vi "Setup Log.vi"(0 "reference in":refnum<class "Result Logger.lvclass">, 4 "Logger Save Folder Path":path, 5 "error in (no error)":errorcluster, 7 "File Column Headers":string[](array[string])) -> (14 "reference out":refnum<class "Result Logger.lvclass">, 19 "error out":errorcluster)   [LabVIEW 2017, in "Result Logger.lvclass"]
uses:
  Result Logger.lvclass
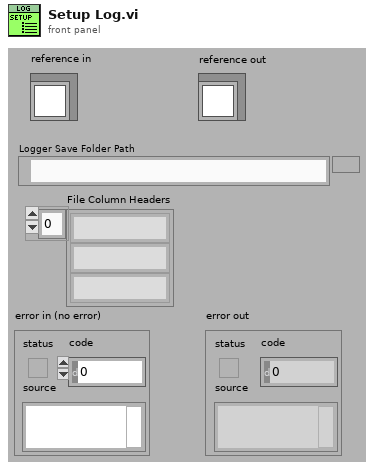
[diagram p1: front panel]
types:
  T1 = enum16{"open", "replace", "create", "open or create", "replace or create", "replace or create with confirmation"}
  T2 = typedef "Result Logger.lvclass/ObjectAttributes.ctl" = cluster{"Logger File Path":path, "Logger File Stream":refnum<file>, "Log Messages":T3[]}
  T3 = typedef "Result Logger.lvclass/Message.ctl" = cluster{"UUT Info":cluster{"Part Number":string, "Lower Push Limit (lb)":dbl, "Upper Push Limit (lb)":dbl, "Lower Pull Limit (lb)":dbl, "Upper Pull Limit (lb)":dbl, "Push Position (mm)":dbl, "Pull Position (mm)":dbl}, "Test Results":cluster{"Test Time":timestamp, "Number of Trials":u32, "Push Values (lb)":dbl[], "Push Average (lb)":dbl, "Push Std Dev (lb)":dbl, "Push Passed":bool, "Pull Values (lb)":dbl[], "Pull Average (lb)":dbl, "Pull Std Dev (lb)":dbl, "Pull Passed":bool}}
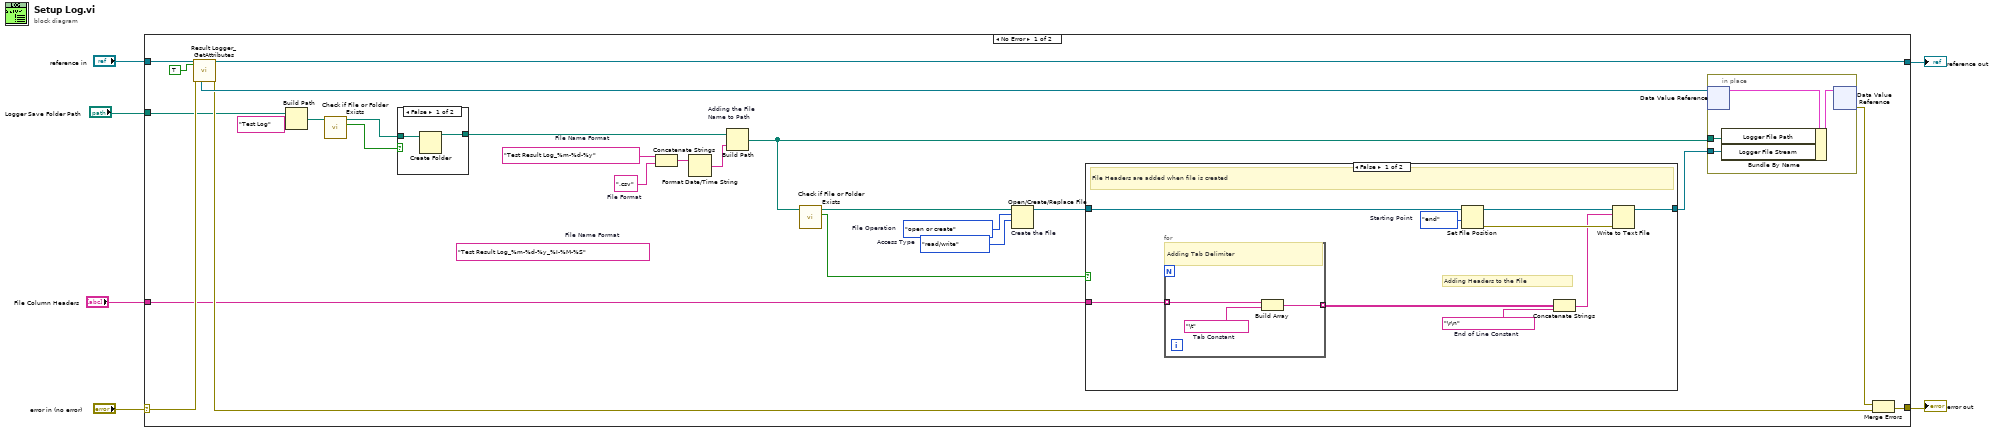
[diagram p0: block diagram]
diagram:
  n1 = case shown="No Error" "error in (no error)" {
    selector: "error in (no error)" -> [w29 w54]
    tunnel: [w31 w54] -> w5
    tunnel: [w27 w53] -> w3
    tunnel: "reference in" -> [w30 w53]
    tunnel: "Logger Save Folder Path" -> [w16 _]
    tunnel: "File Column Headers" -> [w7 _]
    frame No Error {
      w10 = T1."open or create"  # File Operation
      w11 = enum16{"read/write", "read-only", "write-only"}."read/write"  # Access Type
      w14 = "Test Result Log_%m-%d-%y"  # File Name Format
      w22 = ".csv"  # File Format
      (unwired) "Test Result Log_%m-%d-%y_%I-%M-%S"  # File Name Format
      n2 = call "Result Logger_GetAttributes.vi"("reference in"=w30, "OnlyGetDvrReference(False)"=TRUE, "error in (no error)"=w29) -> ("reference out"=w27:refnum<class "Result Logger.lvclass">, "DataRef"=w28:refnum<data-value>, "error out"=w20:errorcluster)  [unwired: 13 in, 1 out]
      n3 = Build Path(base path=w16, name or relative path="Test Log") -> (appended path=w17:path)
      n4 = call <vilib>:"Check if File or Folder Exists.vi"("path"=w17) -> ("file or folder exists?"=w25:bool, "dup path"=w19:path)  [unwired: 8 in, 1 out]
      n5 = case shown="False" w25 {
        tunnel: [w34 w35] -> w21
        tunnel: w19 -> [w33 w35]
        frame False {
          n6 = Create Folder(path (use dialog)=w33) -> (created path=w34:path)  [unwired: 2 in, 2 out]
        }
        frame True {
        }
      }
      n7 = Concatenate Strings(w14, w22) -> (w24:string)
      n8 = Format Date/Time String(time format string (%c)=w24) -> (date/time string=w23:string)  [unwired: 2 in]
      n9 = Build Path "Adding the File \nName to Path"(base path=w21, name or relative path=w23) -> (appended path=w13:path)
      n10 = call <vilib>:"Check if File or Folder Exists.vi"("path"=w13) -> ("file or folder exists?"=w12:bool, "dup path"=w8:path)  [unwired: 8 in, 1 out]
      n11 = Open/Create/Replace File "Create the File"(file path (use dialog)=w8, operation (0:open)=w10, access (0:read/write)=w11) -> (refnum out=w9:refnum<file>)  [unwired: 3 in, 2 out]
      n12 = case shown="False" w12 {
        tunnel: [w41 w48] -> w15
        tunnel: w9 -> [w39 w48]
        tunnel: w7 -> [w37 _]
        frame False {
          w42 = enum16{"start", "end", "current"}."end"  # Starting Point
          w38 = "\r\n"  # End of Line Constant
          # "Adding Headers to the File"
          # "File Headers are added when file is created"
          n13 = for {
            tunnel: w37 -> [w47] mode=indexing
            tunnel: [w45] -> w36 mode=indexing
            w46 = "\t"  # Tab Constant
            # "Adding Tab Delimiter"
            n14 = Build Array(w47, w46) -> (w45:string[])
          }
          n15 = Set File Position(refnum=w39, from (0:start)=w42) -> (refnum out=w44:refnum<file>, error out=w43:errorcluster)  [unwired: 2 in]
          n16 = Concatenate Strings(w36, w38) -> (w40:string)
          n17 = Write to Text File(file (use dialog)=w44, text=w40, error in=w43) -> (refnum out=w41:refnum<file>)  [unwired: 1 in, 2 out]
        }
        frame True {
        }
      }
      n18 = in-place {
        in-place-border: w13 -> [w50]
        in-place-border: w15 -> [w49]
        n19 = in-place-dvr #1(w28) -> (w51:T2)  [unwired: 1 out]
        n20 = Bundle By Name(cluster=w51, "Logger File Path"=w50, "Logger File Stream"=w49) -> (w52:T2)
        n21 = in-place-dvr #1(w52) -> (w32:errorcluster)  [unwired: 1 out]
      }
      n22 = Merge Errors(w32, w20) -> (w31:errorcluster)
    }
    frame Error {
    }
  }
  "error out" <- w5
  "reference out" <- w3
